vi "Open Server Connection.vi"(8 "error in (no error)":errorcluster, 9 "Port":u16, 10 "address":string, 11 "RemoteControl.ZMQ in":refnum<class "RemoteControl.ZMQ.lvclass">) -> (0 "error out":errorcluster, 3 "RemoteControl.ZMQ out":refnum<class "RemoteControl.ZMQ.lvclass">)   [LabVIEW 2019, in "RemoteControl.ZMQ.lvclass"]
uses:
  RemoteControl.ZMQ.lvclass
  <vilib>/addons/zeromq/socket_type.ctl
  RemoteControl.ZMQ.lvclass/RemoteControl.ZMQ.ctl
  <vilib>/addons/zeromq/zmq_context.lvclass
  <vilib>/addons/zeromq/zmq_socket.lvclass
  <vilib>/addons/zeromq/zeromq.lvlib
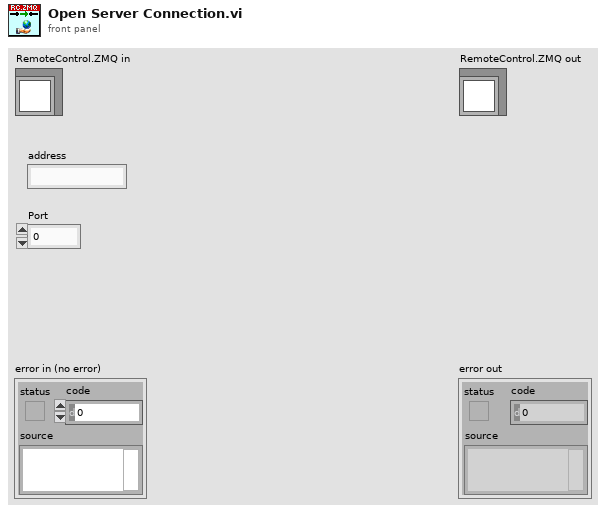
[diagram p1: front panel]
types:
  T1 = typedef "zeromq.lvlib/socket_type.ctl" = enum8{"ZMQ_PAIR", "ZMQ_PUB", "ZMQ_SUB", "ZMQ_REQ", "ZMQ_REP", "ZMQ_DEALER", "ZMQ_ROUTER", "ZMQ_PULL", "ZMQ_PUSH", "ZMQ_XPUB", "ZMQ_XSUB"}
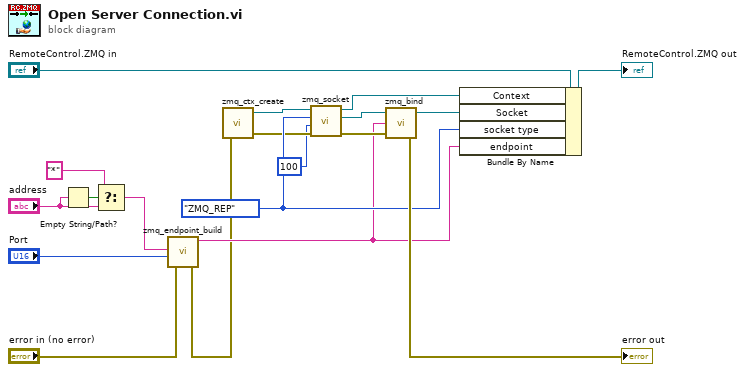
[diagram p0: block diagram]
diagram:
  w14 = socket_type."ZMQ_REP" ("socket type")
  n1 = Empty String/Path?(string/path="address") -> (empty?=w10:bool)
  n2 = Select(t="*", s=w10, f="address") -> (s? t:f=w7:string)
  n3 = call <vilib>:"zmq_endpoint_build.vi"("error in"="error in (no error)", "port"="Port", "address"=w7) -> ("error out"=w3:errorcluster, "endpoint"=w11:string)  [unwired: 2 in, 1 out]
  n4 = call <vilib>:"zmq_ctx_create.vi"("error in"=w3) -> ("error out"=w2:errorcluster, "context out"=w4:refnum<class "zmq_context.lvclass">)  [unwired: 3 in]
  n5 = call <vilib>:"zmq_socket.vi"("error in"=w2, "linger (ms)"=100, "socket type"=w14, "context in"=w4) -> ("error out"=w17:errorcluster, "socket out"=w18:refnum<class "zmq_socket.lvclass">, "context out"=w5:refnum<class "zmq_context.lvclass">)  [unwired: 1 in]
  n6 = call <vilib>:"zmq_bind.vi"("error in"=w17, "endpoint"=w11, "socket in"=w18) -> ("error out"=→"error out":errorcluster, "socket out"=w15:refnum<class "zmq_socket.lvclass">)  [unwired: 1 in]
  n7 = Bundle By Name(cluster="RemoteControl.ZMQ in", "Context"=w5, "Socket"=w15, "socket type"=w14, "endpoint"=w11) -> (→"RemoteControl.ZMQ out":refnum<class "RemoteControl.ZMQ.lvclass">)
